vi "Info to Concatenated String.vi"(9 "Info Array":string[](array[string]), 11 "Title Array":string[](array[string])) -> (3 "Concatenated\nData":string)   [LabVIEW 2013]
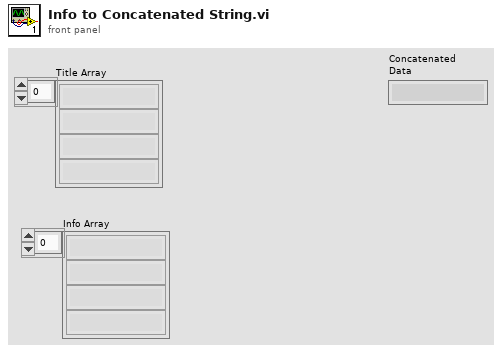
[diagram p1: front panel]
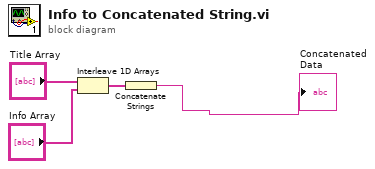
[diagram p0: block diagram]
diagram:
  n1 = Interleave 1D Arrays("Title Array", "Info Array") -> (w4:string[])
  n2 = Concatenate Strings(w4) -> (→"Concatenated\nData":string)
